vi "readInXml.vi"(8 "error in (no error)":errorcluster, 10 "Path":path, 11 "PixelflySettings in":refnum<class "PixelflySettings.lvclass">) -> (0 "error out":errorcluster, 3 "PixelflySettings out":refnum<class "PixelflySettings.lvclass">)   [LabVIEW 2011, in "Tools.lvlib" / "Settings.lvlib" / "PixelflySettings.lvclass"]
uses:
  PixelflySettings.lvclass
  NativeXML/NativeXML.lvclass
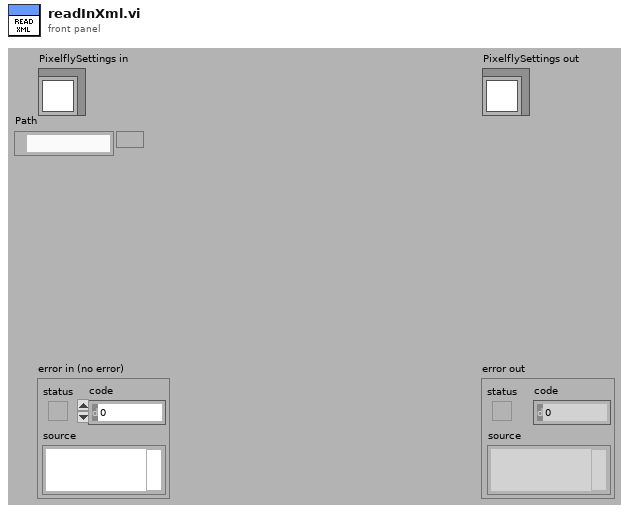
[diagram p1: front panel]
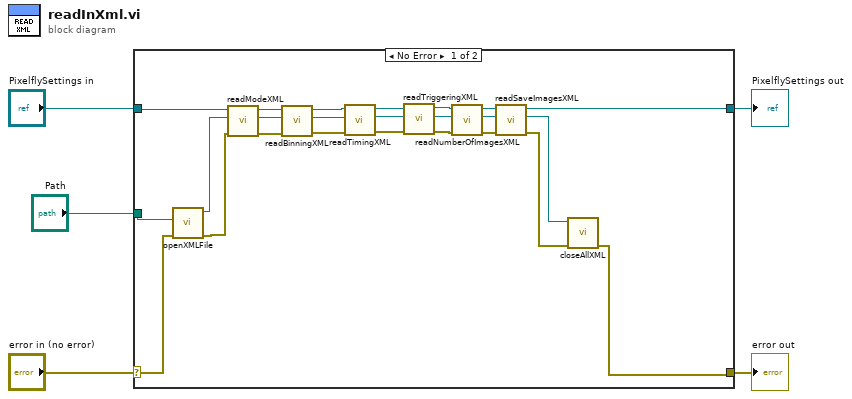
[diagram p0: block diagram]
diagram:
  n1 = case shown="No Error" "error in (no error)" {
    selector: "error in (no error)" -> [w28 w31]
    tunnel: [w15 w31] -> w4
    tunnel: [w7 w30] -> w2
    tunnel: "PixelflySettings in" -> [w27 w30]
    tunnel: "Path" -> [w29 _]
    frame No Error {
      n2 = call "openXMLFile.vi"("error in (no error)"=w28, "Path"=w29) -> ("error out"=w25:errorcluster, "NativeXML out"=w26:refnum<class "NativeXML.lvclass">)  [unwired: 8 in]
      n3 = call "readModeXML.vi"("error in (no error)"=w25, "NativeXML in"=w26, "PixelflySettings in"=w27) -> ("error out"=w22:errorcluster, "NativeXML out"=w23:refnum<class "NativeXML.lvclass">, "PixelflySettings out"=w24:refnum<class "PixelflySettings.lvclass">)  [unwired: 6 in]
      n4 = call "readBinningXML.vi"("error in (no error)"=w22, "NativeXML in"=w23, "PixelflySettings in"=w24) -> ("error out"=w20:errorcluster, "NativeXML out"=w19:refnum<class "NativeXML.lvclass">, "PixelflySettings out"=w21:refnum<class "PixelflySettings.lvclass">)  [unwired: 6 in]
      n5 = call "readTimingXML.vi"("error in (no error)"=w20, "NativeXML in"=w19, "PixelflySettings in"=w21) -> ("error out"=w17:errorcluster, "NativeXML out"=w16:refnum<class "NativeXML.lvclass">, "PixelflySettings out"=w18:refnum<class "PixelflySettings.lvclass">)  [unwired: 6 in]
      n6 = call "readTriggeringXML.vi"("error in (no error)"=w17, "NativeXML in"=w16, "PixelflySettings in"=w18) -> ("error out"=w12:errorcluster, "NativeXML out"=w13:refnum<class "NativeXML.lvclass">, "PixelflySettings out"=w14:refnum<class "PixelflySettings.lvclass">)  [unwired: 6 in]
      n7 = call "readNumberOfImagesXML.vi"("error in (no error)"=w12, "NativeXML in"=w13, "PixelflySettings in"=w14) -> ("error out"=w9:errorcluster, "NativeXML out"=w10:refnum<class "NativeXML.lvclass">, "PixelflySettings out"=w11:refnum<class "PixelflySettings.lvclass">)  [unwired: 6 in]
      n8 = call "readSaveImagesXML.vi"("error in (no error)"=w9, "NativeXML in"=w10, "PixelflySettings in"=w11) -> ("error out"=w8:errorcluster, "NativeXML out"=w6:refnum<class "NativeXML.lvclass">, "PixelflySettings out"=w7:refnum<class "PixelflySettings.lvclass">)  [unwired: 6 in]
      n9 = call "closeAllXML.vi"("error in (no error)"=w8, "NativeXML in"=w6) -> ("error out"=w15:errorcluster)  [unwired: 9 in]
    }
    frame Error {
    }
  }
  "error out" <- w4
  "PixelflySettings out" <- w2
